vi "FTW-Message-Request-Interpret.vi"(8 "error in":errorcluster, 11 "FTW Incoming Request":refnum<class "FTW-Message-HttpRequest.lvclass">) -> (0 "error out":errorcluster, 1 "Request Body":string, 2 "Request Header":string, 3 "FTW Incoming Request out":refnum<class "FTW-Message-HttpRequest.lvclass">)   [LabVIEW 2015, in "FTW-Message-HttpRequest.lvclass"]
uses:
  FTW-Message-HttpRequest.lvclass
panel:
  # "Inputs"
  # "Outputs"
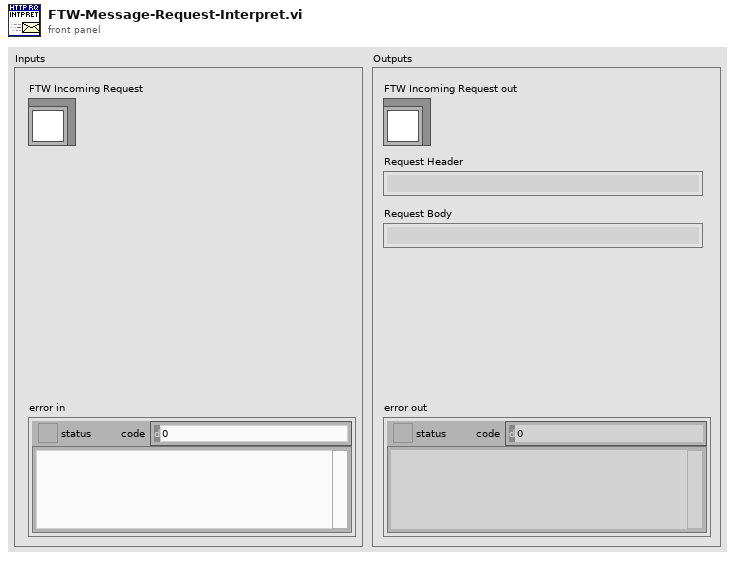
[diagram p1: front panel]
types:
  T1 = typedef "FTW-MessagePayload.ctl" = cluster{"Header":string, "Body":string, "FTW: Sender Identity":string, "FTW: Reply Address":string, "FTW: Reply Error":errorcluster}
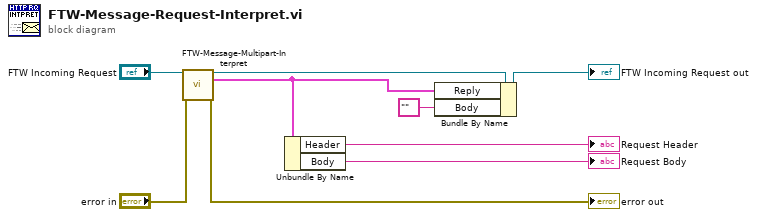
[diagram p0: block diagram]
diagram:
  n1 = call-dynamic "FTW-Message-Multipart-Interpret.vi"("FTW Message"="FTW Incoming Request", "error in"="error in") -> ("FTW Message out"=w8:refnum<class "FTW-Message-HttpRequest.lvclass">, "Message"=w2:T1, "error out"=→"error out":errorcluster)  [unwired: 11 in]
  n2 = Unbundle By Name(w2) -> ("Header"=→"Request Header":string, "Body"=→"Request Body":string)
  n3 = Bundle By Name(cluster=w8, "Reply"=w2, "Body"="" ("empty string")) -> (→"FTW Incoming Request out":refnum<class "FTW-Message-HttpRequest.lvclass">)
